vi "GA_Select Parent.vi"(6 "Parameters":T1={"Population size"=100, "Generations no."=500, "Crossover probabality"=6.0, "Mutation mode"=enum."one-point, fitness-adjustable rate", "Creep mutation"=FALSE, "Mutation rate"=0.005, "Min mutation rate"=0.005, "Max mutation rate"=0.0005, "Relative fitness differential"=0.25, "Reproduction plan"=enum."Steady-state-replace-random", "Elitism"=FALSE, "FeaturesPerChannel"=0} {"Relative fitness differential" min=0.0 max=1.0; "Max mutation rate" min=0.0 max=1.0; "Min mutation rate" min=0.0 max=1.0; "Mutation rate" min=0.0 max=1.0; "Crossover probabality" min=0.0 max=1.0; "Generations no." min=1; "Population size" min=1}, 11 "Ranks":i32[](array[numeric])) -> (3 "Parent index":i32)   [LabVIEW 2016, in "GA.lvlib"]
doc: "Selects one parent from population. For higher \"Relative fitness differencial\" (0-1) more likely better individuals become parents."
uses:
  GA.lvlib
  GA_tParameters.ctl
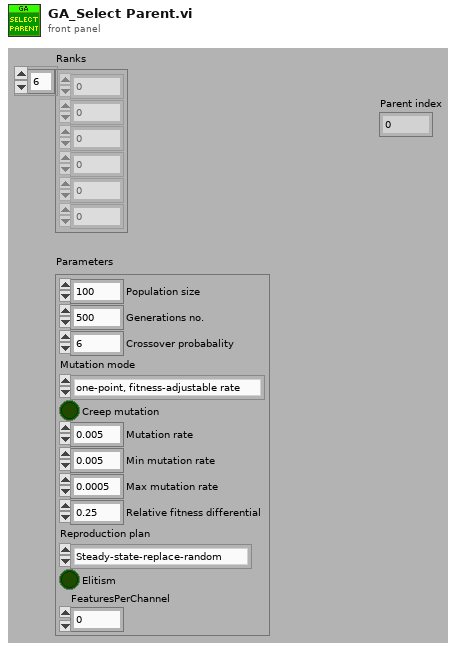
[diagram p1: front panel]
types:
  T1 = typedef "GA.lvlib/GA_tParameters.ctl" = cluster{"Population size":i32, "Generations no.":i32, "Crossover probabality":dbl, "Mutation mode":enum16{"one-point, fixed rate", "one-point, fitness-adjustable rate", "one-point, distance-adjustable rate"}, "Creep mutation":bool, "Mutation rate":dbl, "Min mutation rate":dbl, "Max mutation rate":dbl, "Relative fitness differential":dbl, "Reproduction plan":enum16{"Full generational replacement", "Steady-state-replace-random", "Steady-state-replace-worst"}, "Elitism":bool, "FeaturesPerChannel":i32}
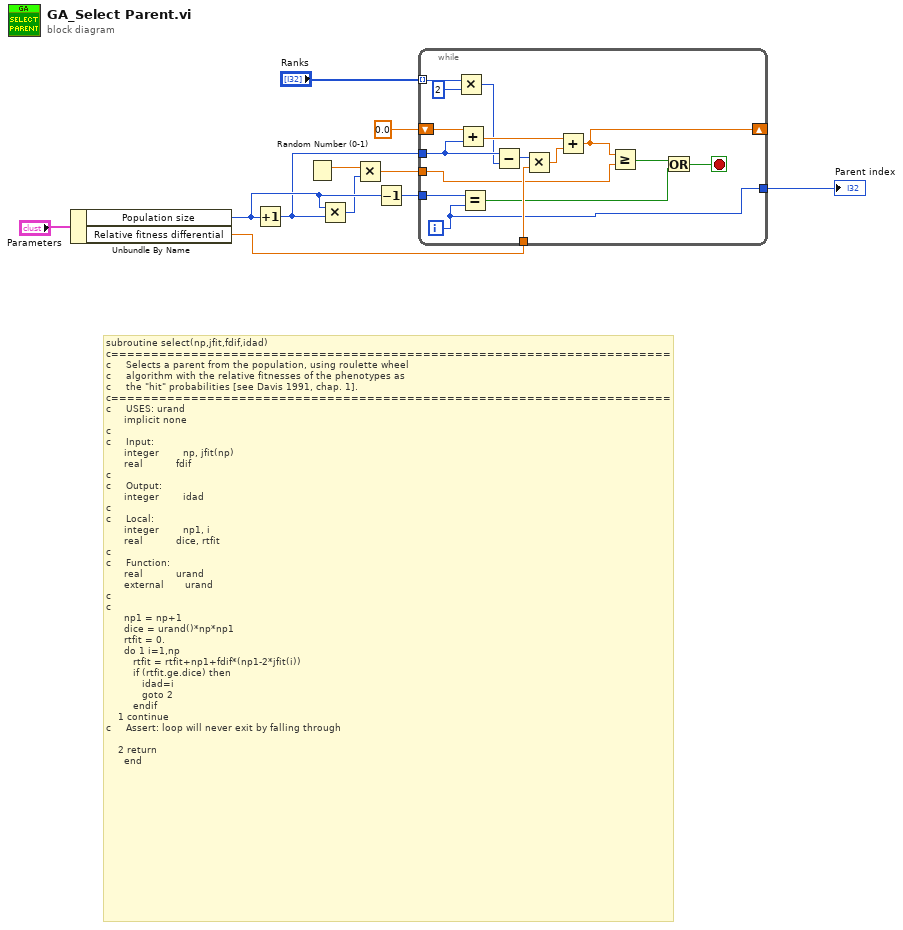
[diagram p0: block diagram]
diagram:
  # "subroutine select(np,jfit,fdif,idad)\nc======================================================================\nc     Selects a parent from the population, using roulette wheel\nc     algorithm with the relative fitnesses of the phenotypes as\nc     the \"hit\" probabilities [see Davis 1991, chap. 1].\nc======================================================================\nc     USES: urand\n      implicit none\nc\nc     Input:\n      integer        np, jfit(np)\n      real           fdif\nc\nc     Output:\n      integer        idad\nc\nc     Local:\n      integer        np1, i\n      real           dice, rtfit\nc\nc     Function:\n      real           urand\n      external       urand\nc\nc\n      np1 = np+1\n      dice = urand()*np*np1\n      rtfit = 0.\n      do 1 i=1,np\n         rtfit = rtfit+np1+fdif*(np1-2*jfit(i))\n         if (rtfit.ge.dice) then\n            idad=i\n            goto 2\n         endif\n    1 continue\nc     Assert: loop will never exit by falling through\n \n    2 return\n      end"
  n1 = Unbundle By Name("Parameters") -> ("Population size"=w8:i32, "Relative fitness differential"=w11:dbl)
  n2 = Increment(x=w8) -> (x+1=w2:i32)
  n3 = Random Number (0-1)() -> (number: 0 to 1=w7:dbl)
  n4 = Multiply(x=w8, y=w2) -> (x*y=w6:i32)
  n5 = Multiply(x=w7, y=w6) -> (x*y=w4:dbl)
  n6 = Decrement(x=w8) -> (x-1=w1:i32)
  n7 = while {
    tunnel: "Ranks" -> [w12] mode=indexing
    tunnel: w1 -> [w27]
    tunnel: w4 -> [w18]
    shift-right: [w19] -> _
    shift-left: 0.0 -> [w26]
    tunnel: w2 -> [w24]
    tunnel: w11 -> [w22]
    tunnel: [w13] -> w9
    i -> [w13]
    stop <- w15 stop-if-true
    n8 = Multiply(x=w12, y=2) -> (x*y=w14:i32)
    n9 = Add(x=w26, y=w24) -> (x+y=w21:dbl)
    n10 = Equal?(x=w27, y=w13) -> (x = y?=w16:bool)
    n11 = Subtract(x=w24, y=w14) -> (x-y=w23:i32)
    n12 = Multiply(x=w23, y=w22) -> (x*y=w20:dbl)
    n13 = Add(x=w21, y=w20) -> (x+y=w19:dbl)
    n14 = Greater Or Equal?(x=w19, y=w18) -> (x >= y?=w17:bool)
    n15 = Or(x=w17, y=w16) -> (x .or. y?=w15:bool)
  }
  "Parent index" <- w9
